vi "Do Action.vi"(8 "error in (no error)":errorcluster, 9 "Display Queue":refnum<queue>, 10 "tlc_User Event Reference.ctl":T1, 11 "Save in":refnum<class "Save.lvclass">) -> (0 "error out":errorcluster)   [LabVIEW 2010, in "Save.lvclass"]
doc: "This instance of Do Action.vi is used to perform the functionality that was previously contained in the Save case of the consumer loop.\n\nThis method will save the current cue list to a file that can be loaded later."
uses:
  Save.lvclass
  Controls/tlc_User Interface Command.ctl
  Controls/tlc_User Interface Data Type.ctl
  Controls/tlc_User Event Reference.ctl
  Modules/Cue/tlc_Cue_Information Command.ctl
  Modules/File/tlc_File_Command Control.ctl
  Save.lvclass/Save.ctl
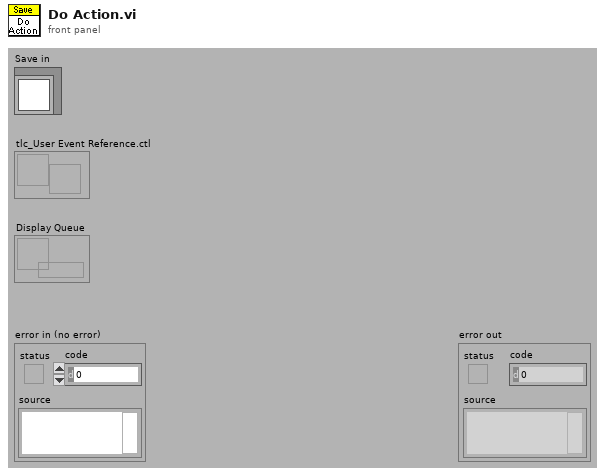
[diagram p1: front panel]
types:
  T1 = typedef "tlc_User Event Reference.ctl" = refnum<user-event>
  T2 = typedef "tlc_File_Command Control.ctl" = enum16{"Initialize", "Save Cues", "Load Cues", "Shutdown"}
  T3 = typedef "tlc_Cue_Information Command.ctl" = enum16{"Add Cue", "Get Cue Values", "Set Cue Values", "Get Number of Cues", "Initialize", "Get Empty Cue"}
  T4 = typedef "tlc_Cue_Information.ctl" = cluster{"Cue Name":string, "Wait Time (s)":u32, "Fade Time (s)":u32, "Follow Time (s)":u32, "Channels":T5[][]}
  T5 = typedef "channel.ctl" = cluster{"Intensity":dbl, " Color":u32, "Channel":i32}
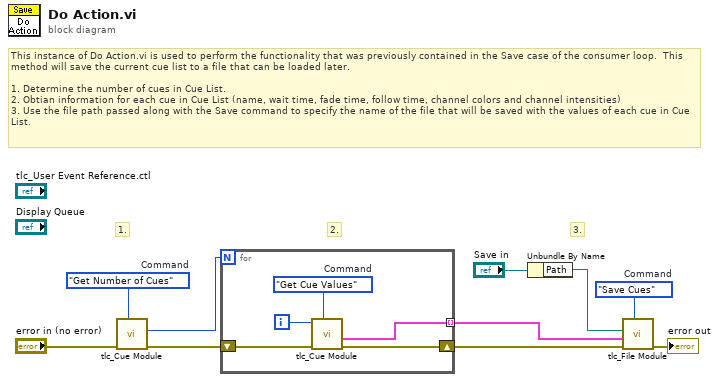
[diagram p0: block diagram]
diagram:
  w10 = tlc_File_Command_Control."Save Cues"  # Command
  w5 = tlc_Cue_Information_Command."Get Number of Cues"  # Command
  # "3."
  # "2."
  # "1."
  # "This instance of Do Action.vi is used to perform the functionality that was previously contained in the Save case of the consumer loop.  This method will save the current cue list to a file that can be loaded later.\n\n1. Determine the number of cues in Cue List.\n2. Obtian information for each cue in Cue List (name, wait time, fade time, follow time, channel colors and channel intensities)\n3. Use the file path passed along with the Save command to specify the name of the file that will be saved with the values of each cue in Cue List."
  n1 = call "tlc_Cue Module.vi"("Command"=w5, "error in (no error)"="error in (no error)") -> ("error out"=w7:errorcluster, "Number of Cues"=w6:i32)  [unwired: 6 in, 1 out]
  n2 = for {
    N: w6 -> [_]
    shift-right: [w14] -> w8
    shift-left: w7 -> [w15]
    tunnel: [w13] -> w9 mode=indexing
    i -> [w12]
    w11 = tlc_Cue_Information_Command."Get Cue Values"  # Command
    n3 = call "tlc_Cue Module.vi"("Command"=w11, "error in (no error)"=w15, "Cue Index"=w12) -> ("error out"=w14:errorcluster, "Cue Output"=w13:T4)  [unwired: 5 in, 1 out]
  }
  n4 = Unbundle By Name "Unbundle By Name"("Save in") -> ("Path"=w1:path)
  n5 = call "tlc_File Module.vi"("Command"=w10, "error in (no error)"=w8, "Cue Array Input"=w9, "Path"=w1) -> ("error out"=→"error out":errorcluster)  [unwired: 6 in, 1 out]
